vi "Find Label References.vi"(0 "item ref in":T1 format="%.0x", 5 "decimalLabel":i32, 7 "SDI enabled":bool, 9 "SDI value":u8, 11 "error in":errorcluster) -> (4 "Array of Refs":T1[](array[typedef]) format="%.0x", 6 "Found":bool, 15 "error out":errorcluster)   [LabVIEW 2020, in "Communication Bus Template Scripting.lvlib"]
uses:
  <vilib>/NI VeriStand/Custom Device API/Custom Device Item Ref.ctl
  Constants.vi
  <vilib>/NI VeriStand/Custom Device API/Get Item Property (U32).vi
  <vilib>/NI VeriStand/Custom Device API/Get Item Property (Boolean).vi
  Communication Bus Template Scripting.lvlib
  <vilib>/NI VeriStand/Custom Device API/Custom Device API.lvlib
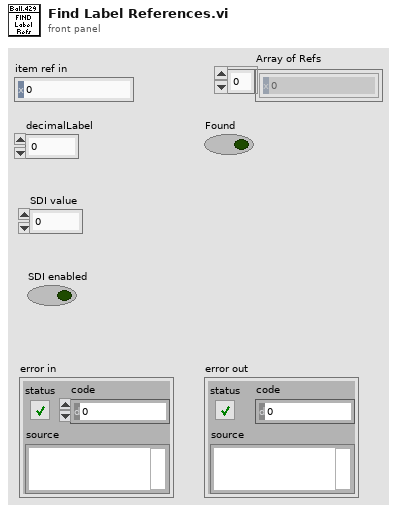
[diagram p1: front panel]
types:
  T1 = typedef "Custom Device API.lvlib/Custom Device Item Ref.ctl" = u64
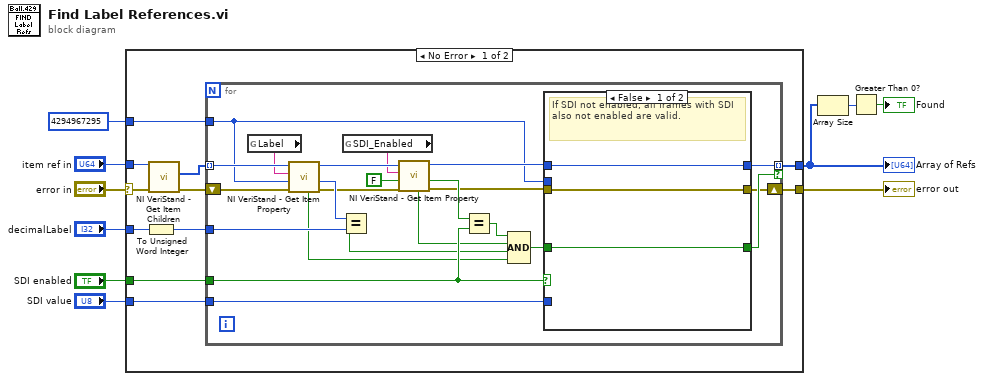
[diagram p0: block diagram]
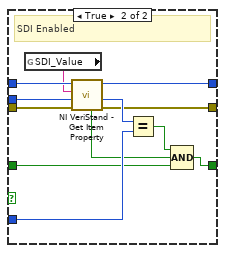
[diagram p2: hidden frame]
diagram:
  n1 = case shown="No Error" "error in" {
    selector: "error in" -> [w17 w60]
    tunnel: "decimalLabel" -> [w21 _]
    tunnel: [w20 w60] -> w9
    tunnel: "item ref in" -> [w19 _]
    tunnel: [w14 _] -> w6
    tunnel: "SDI value" -> [w13 _]
    tunnel: "SDI enabled" -> [w12 _]
    tunnel: u32 4294967295 ("Default Value") -> [w11 _]
    frame No Error {
      n2 = To Unsigned Word Integer(number=w21) -> (unsigned 16bit integer=w16:u16)
      n3 = call <vilib>:"NI VeriStand - Get Item Children.vi"("error in (no error)"=w17, "Item Ref in"=w19) -> ("error out"=w18:errorcluster, "Child Refs"=w15:T1[])  [unwired: 6 in, 2 out]
      n4 = for {
        tunnel: w16 -> [w43]
        shift-right: [w37] -> w20
        shift-left: w18 -> [w44]
        tunnel: w15 -> [w41] mode=indexing
        tunnel: [w39] -> w14 mode=indexing if=w40
        tunnel: w13 -> [w38]
        tunnel: w12 -> [w32]
        tunnel: w11 -> [w29]
        n5 = global read "Constants.vi" "Label"() -> (w23:string)
        n6 = call-poly <vilib>:"NI VeriStand - Get Item Property.vi"("error in (no error)"=w44, "Default Value"=w29, "Property Name"=w23, "Item Ref in"=w41) -> ("error out"=w31:errorcluster, "Value"=w42:u32, "Item Ref out"=w34:T1, "Found?"=w25:bool)  [unwired: 4 in]
        n7 = Equal?(x=w42, y=w43) -> (x = y?=w26:bool)
        n8 = global read "Constants.vi" "SDI_Enabled"() -> (w22:string)
        n9 = call-poly <vilib>:"NI VeriStand - Get Item Property.vi"("error in (no error)"=w31, "Default Value"=FALSE, "Property Name"=w22, "Item Ref in"=w34) -> ("error out"=w30:errorcluster, "Value"=w35:bool, "Item Ref out"=w33:T1, "Found?"=w27:bool)  [unwired: 4 in]
        n10 = Equal?(x=w35, y=w32) -> (x = y?=w28:bool)
        n11 = Compound Arithmetic op=AND(w28, w27, w26, w25) -> (w24:bool)
        n12 = case shown="False" w32 {
          tunnel: [w45 w59] -> w40
          tunnel: w33 -> [w47 w57]
          tunnel: [w47 w56] -> w39
          tunnel: w38 -> [_ w55]
          tunnel: w30 -> [w46 w54]
          tunnel: [w46 w53] -> w37
          tunnel: w29 -> [_ w50]
          tunnel: w24 -> [w45 w49]
          frame False {
            # "If SDI not enabled, all frames with SDI also not enabled are valid."
          }
          frame True {
            # "SDI Enabled"
            n13 = global read "Constants.vi" "SDI_Value"() -> (w48:string)
            n14 = call-poly <vilib>:"NI VeriStand - Get Item Property.vi"("error in (no error)"=w54, "Default Value"=w50, "Property Name"=w48, "Item Ref in"=w57) -> ("error out"=w53:errorcluster, "Value"=w58:u32, "Item Ref out"=w56:T1, "Found?"=w52:bool)  [unwired: 4 in]
            n15 = Equal?(x=w58, y=w55) -> (x = y?=w51:bool)
            n16 = Compound Arithmetic op=AND(w51, w52, w49) -> (w59:bool)
          }
        }
      }
    }
    frame Error {
    }
  }
  "error out" <- w9
  "Array of Refs" <- w6
  n17 = Array Size(array=w6) -> (size(s)=w5:i32)
  n18 = Greater Than 0?(x=w5) -> (x > 0?=→"Found":bool)
